vi "G_init.vi"(10 "G":i32[](array[numeric]), 11 "Initialization":T1) -> (3 "G(out)":dbl[](array[numeric]))   [LabVIEW 2014]
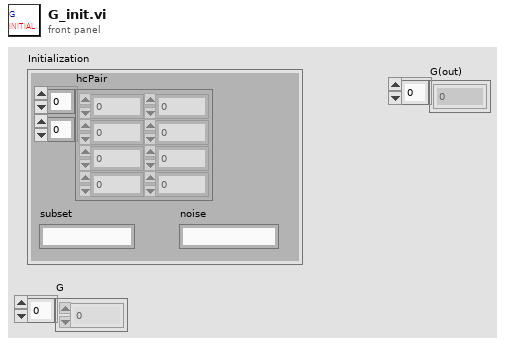
[diagram p1: front panel]
types:
  T1 = cluster{"subset":string, "noise":string, "hcPair":dbl[][]}
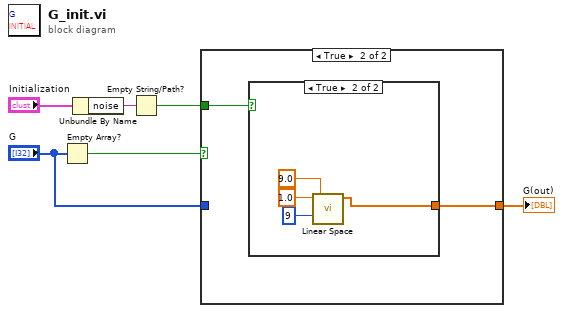
[diagram p0: block diagram]
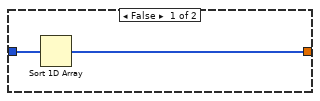
[diagram p2: hidden frame]
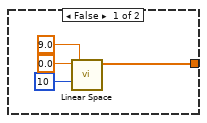
[diagram p3: hidden frame]
diagram:
  n1 = Empty Array?(array="G") -> (empty?=w5:bool)
  n2 = Unbundle By Name("Initialization") -> ("noise"=w6:string)
  n3 = Empty String/Path?(string/path=w6) -> (empty?=w4:bool)
  n4 = case shown="True" w5 {
    tunnel: w4 -> [_ w10]
    tunnel: "G" -> [w8 _]
    tunnel: [w7 w9] -> w2
    frame False {
      n5 = Sort 1D Array(array=w8) -> (sorted array=w7:i32[])
    }
    frame True {
      n6 = case shown="True" w10 {
        tunnel: [w11 w15] -> w9
        frame False {
          n7 = call "Linear Space.vi"("Number of Samples"=u32 10, "Maximum"=9.0, "Minimum"=0.0) -> ("Array"=w11:dbl[])  [unwired: 3 in, 1 out]
        }
        frame True {
          n8 = call "Linear Space.vi"("Number of Samples"=u32 9, "Maximum"=9.0, "Minimum"=1.0) -> ("Array"=w15:dbl[])  [unwired: 3 in, 1 out]
        }
      }
    }
  }
  "G(out)" <- w2
